vi "Forward Debug Data to Handler.vi"(8 "error in (no error)":errorcluster, 10 "Debug Data Cluster":refnum<class "Debug Data.lvclass">, 11 "Debug Message Receiver In":refnum<class "Debug Message Receiver.lvclass">) -> (0 "error out":errorcluster, 3 "Debug Message Receiver Out":refnum<class "Debug Message Receiver.lvclass">)   [LabVIEW 2020, in "Debug Message Receiver.lvclass"]
uses:
  Debug Message Receiver.lvclass
  Debug Data/Debug Data.lvclass
  Debug Message Receiver.lvclass/Debug Message Receiver.ctl
  Debug Data Event/Debug Data Listener.lvclass
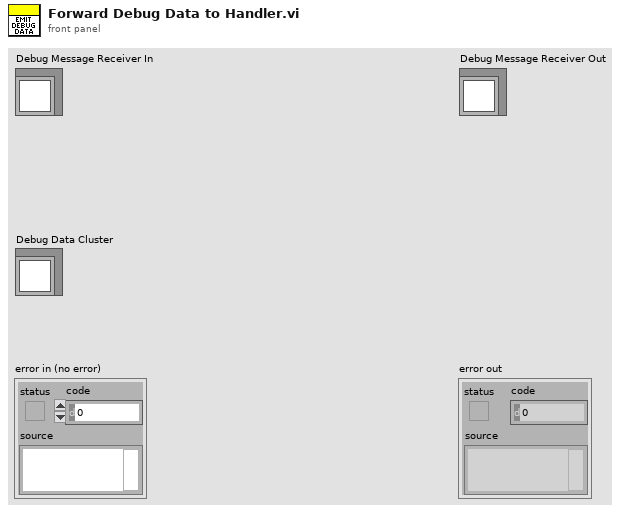
[diagram p1: front panel]
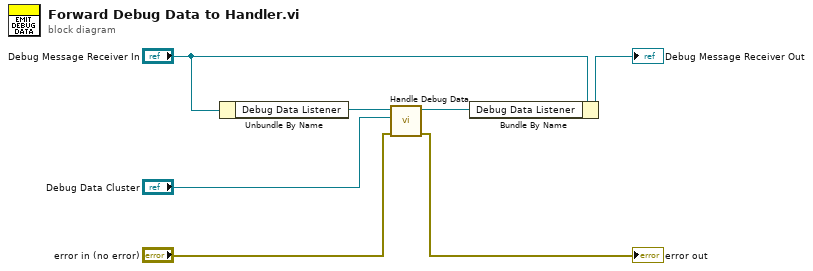
[diagram p0: block diagram]
diagram:
  n1 = Unbundle By Name("Debug Message Receiver In") -> ("Debug Data Listener"=w7:refnum<class "Debug Data Listener.lvclass">)
  n2 = call-dynamic "Handle Debug Data.vi"("error in (no error)"="error in (no error)", "Debug Data.lvclass"="Debug Data Cluster", "Debug Data Event In"=w7) -> ("error out"=→"error out":errorcluster, "Debug Data Event Out"=w1:refnum<class "Debug Data Listener.lvclass">)  [unwired: 7 in]
  n3 = Bundle By Name(cluster="Debug Message Receiver In", "Debug Data Listener"=w1) -> (→"Debug Message Receiver Out":refnum<class "Debug Message Receiver.lvclass">)
